vi "178-malformedtimeAttribute.vi"(8 "error in":errorcluster) -> (0 "error out":errorcluster)   [LabVIEW 2013]
uses:
  classes/Test Report.JUnit/Test Report.JUnit.lvclass
  classes/Test Result/Test Result.lvclass
  classes/Test Result/Assert Event Data (Extended).ctl
  classes/Assert/Assert Equal Value_Variant.vi
  classes/Test Report/Test Report.lvclass
  classes/Assert/Assert.lvclass
  classes/Test/Test.lvclass
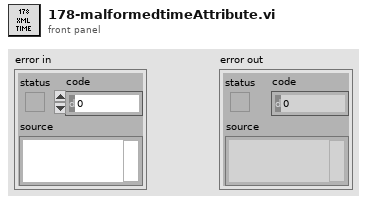
[diagram p1: front panel]
types:
  T1 = typedef "Caraya.lvlib/Test Result.lvclass/Assert Event Data (Extended).ctl" = cluster{"name":string, "passed":bool, "call-chain":string[], "test-error":errorcluster, "timestamp":timestamp, "assert-id":string, "test-id":string, "time":dbl, "message":string, "properties":variant, "measurements":variant, "user-defined":variant}
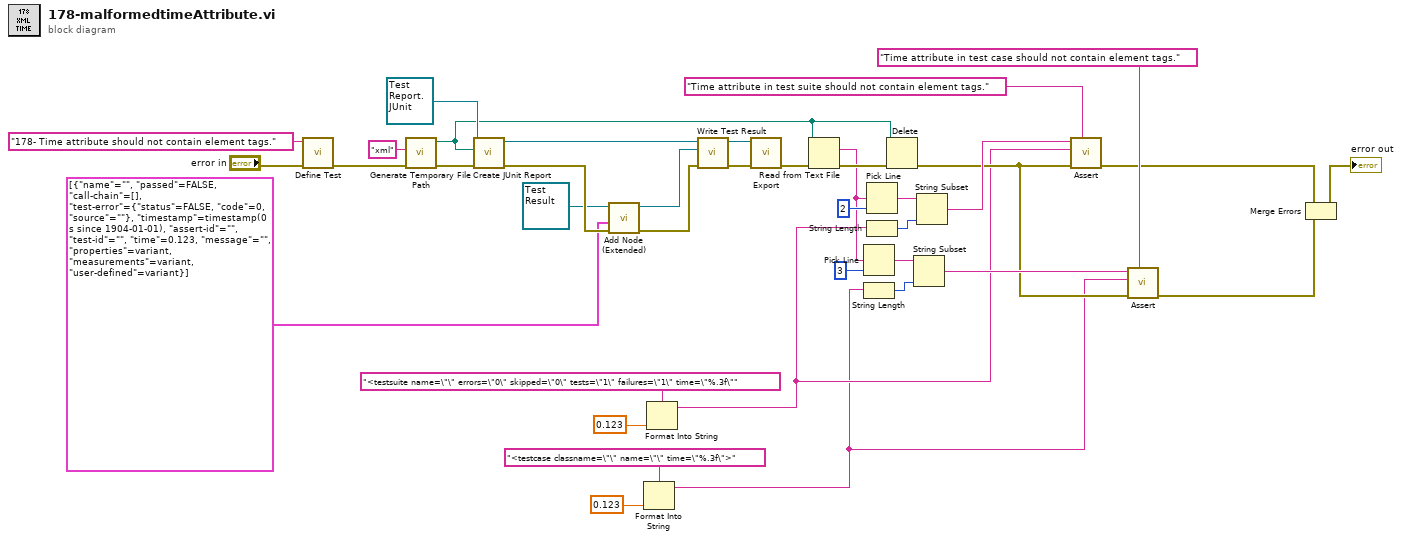
[diagram p0: block diagram]
diagram:
  n1 = call "Define Test.vi"("error in (no error)"="error in", "Label (VI Title)"="178- Time attribute should not contain element tags.") -> ("error out"=w29:errorcluster)  [unwired: 8 in, 1 out]
  n2 = call <vilib>:"Generate Temporary File Path.vi"("error in (no error)"=w29, "Temporary File Extension (tmp)"="xml") -> ("error out"=w33:errorcluster, "Unique Temporary File Path"=w30:path)  [unwired: 8 in]
  n3 = call "Create JUnit Report.vi"("error in (no error)"=w33, "Report Path"=w30, "Test Report.JUnit in"=refnum<class "Test Report.JUnit.lvclass"> refnum) -> ("error out"=w20:errorcluster, "Test Report.JUnit out"=w37:refnum<class "Test Report.JUnit.lvclass">)  [unwired: 7 in]
  n4 = call "Add Node (Extended).vi"("error in (no error)"=w20, "Assertions"=T1[] [{"name"="", "passed"=FALSE, "call-chain"=[], "test-error"={"status"=FALSE, "code"=0, "source"=""}, "timestamp"=timestamp(0 s since 1904-01-01), "assert-id"="", "test-id"="", "time"=0.123, "message"="", "properties"=variant, "measurements"=variant, "user-defined"=variant}], "Test Result in"=refnum<class "Test Result.lvclass"> refnum) -> ("error out"=w21:errorcluster, "Test Result out"=w22:refnum<class "Test Result.lvclass">)  [unwired: 7 in]
  n5 = Format Into String(format string="<testcase classname=\"\" name=\"\" time=\"%.3f\">" ("text"), 0.123 ("time")) -> (resulting string=w2:string)  [unwired: 2 in, 1 out]
  n6 = Format Into String(format string="<testsuite name=\"\" errors=\"0\" skipped=\"0\" tests=\"1\" failures=\"1\" time=\"%.3f\"" ("text"), 0.123 ("time")) -> (resulting string=w6:string)  [unwired: 2 in, 1 out]
  n7 = call "Write Test Result.vi"("error in (no error)"=w21, "Test Result"=w22, "Test Report in"=w37) -> ("error out"=w35:errorcluster, "Test Report out"=w36:refnum<class "Test Report.JUnit.lvclass">)  [unwired: 7 in]
  n8 = call-dynamic "Export.vi"("error in (no error)"=w35, "Test Report in"=w36) -> ("error out"=w32:errorcluster)  [unwired: 8 in, 1 out]
  n9 = Read from Text File(file (use dialog)=w30, error in=w32) -> (text=w12:string, error out=w31:errorcluster)  [unwired: 2 in, 2 out]
  n10 = Pick Line(multi-line string=w12, line index=3) -> (output string=w15:string)  [unwired: 1 in]
  n11 = String Length(string=w2) -> (length=w16:i32)
  n12 = Pick Line(multi-line string=w12, line index=2) -> (output string=w25:string)  [unwired: 1 in]
  n13 = String Length(string=w6) -> (length=w24:i32)
  n14 = Delete(path (use dialog)=w30, error in=w31) -> (error out=w8:errorcluster)  [unwired: 3 in, 2 out]
  n15 = String Subset(string=w15, length (rest)=w16) -> (substring=w13:string)  [unwired: 1 in]
  n16 = String Subset(string=w25, length (rest)=w24) -> (substring=w23:string)  [unwired: 1 in]
  n17 = call-poly "Assert.vi"("Label"="Time attribute in test suite should not contain element tags.", "error in (no error)"=w8, "Y"=w6, "X"=w23) -> ("error out"=w11:errorcluster)  [unwired: 6 in, 1 out]
  n18 = call-poly "Assert.vi"("Label"="Time attribute in test case should not contain element tags.", "error in (no error)"=w8, "Y"=w2, "X"=w13) -> ("error out"=w10:errorcluster)  [unwired: 6 in, 1 out]
  n19 = Merge Errors(w11, w10) -> (→"error out":errorcluster)
